vi "PH_BL-Master.PC calc Vac State.vi"(0 "i ref in":refnum<vi>, 2 "Channel Name":string="N/A", 4 "no link":bool, 5 "error in (no error)":errorcluster) -> (14 "i ref out":refnum<vi>, 19 "error out":errorcluster)   [LabVIEW 2014, in "PH_BL-Master.lvlib"]
doc: "This VI sets the vac state to GUI elements and stores it to own attributes."
uses:
  PH_BL-Master.lvlib
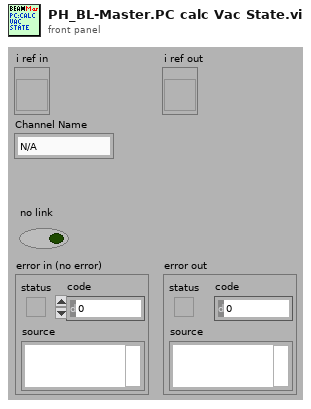
[diagram p1: front panel]
types:
  T1 = typedef "PH_BL-Master.lvlib/PH_BL-Master.i attribute.ctl" = cluster{"Remote controlled":bool, "Boolean Condition Service Subscriber":refnum<vi>[], "Picture Condition Service Subscriber":refnum<vi>[], "R2S":cluster{"GUI Ref":refnum<vi>, "State":bool}, "Vacua":cluster{"GUI Ref":refnum<vi>, "Limit":dbl, "Curr Value":dbl, "in range":bool}[], "O2 Inspection":cluster{"GUI Ref":refnum<vi>, "Concentration":dbl, "State":T2}[], "Boolean Status Service Subscriber":cluster{"GUI Ref":refnum<vi>, "Status":T2, "no Link?":bool, "Status Subscriber Class":T3}[], "Picture Status Service Subscriber":cluster{"GUI Ref":refnum<vi>, "Status":T2, "no Link?":bool, "Status Subscriber Class":T3}[], "6P 4Q Service Subscriber":cluster{"GUI Ref":refnum<vi>, "Selector":T4, "no Link?":bool}[], "Index of latest 6P 4Q changing Instance":i32, "Index of latest Picture Status changing Instance":i32, "Index of latest Boolean Status changing Instance":i32, "Vision ID on same Node":string, "Start Phase over?":bool, "GUI Ref Delete":refnum<vi>}
  T2 = typedef "PH_StatusHandler.lvlib/PH_StatusHandler.Status.ctl" = i16
  T3 = typedef "PH_BL-Master.lvlib/PH_BL-Master.Status Subscriber Class.ctl" = enum16{"unknown", "Switch", "BB", "6P Switch", "Switch GUI", "Switch and 6P State", "Force Sensor"}
  T4 = typedef "PH_4_Pos_Selector.lvlib/PH_4_Pos_Selector.Position Selector.ctl" = u16
  T5 = cluster{"GUI Ref":refnum<vi>, "Limit":dbl, "Curr Value":dbl, "in range":bool}[]
  T6 = cluster{"GUI Ref":refnum<vi>, "Limit":dbl, "Curr Value":dbl, "in range":bool}
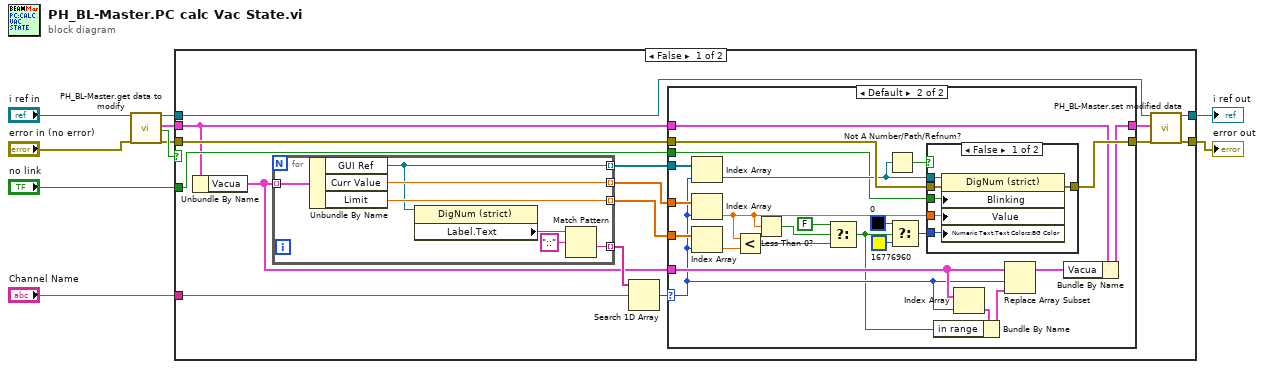
[diagram p0: block diagram]
diagram:
  n1 = call "PH_BL-Master.get data to modify.vi"("i ref in"="i ref in", "error in (no error)"="error in (no error)") -> ("i ref out"=w1:refnum<vi>, "i attribute"=w3:T1, "timed out"=w4:bool, "error out"=w2:errorcluster)  [unwired: 14 in]
  n2 = case shown="False" w4 {
    tunnel: w1 -> [w15 w67]
    tunnel: [w25 w67] -> w9
    tunnel: w2 -> [w23 w66]
    tunnel: [w24 w66] -> w10
    tunnel: w3 -> [w18 _]
    tunnel: "Channel Name" -> [w19 _]
    tunnel: "no link" -> [w21 _]
    frame False {
      n3 = Unbundle By Name(w18) -> ("Vacua"=w14:T5)
      n4 = for {
        tunnel: w14 -> [w65] mode=indexing
        tunnel: [w59] -> w20 mode=indexing
        tunnel: [w64] -> w13 mode=indexing
        tunnel: [w63] -> w12 mode=indexing
        tunnel: [w62] -> w11 mode=indexing
        n5 = Unbundle By Name(w65) -> ("GUI Ref"=w62:refnum<vi>, "Curr Value"=w64:dbl, "Limit"=w63:dbl)
        n6 = property class="DigNum (strict)"(reference=w62) -> ("Label.Text"=w61:string)  [unwired: 1 in, 2 out]
        n7 = Match Pattern(string=w61, regular expression="::") -> (after substring=w59:string)  [unwired: 1 in, 3 out]
      }
      n8 = Search 1D Array(1D array=w20, element=w19) -> (index of element=w16:i32)  [unwired: 1 in]
      n9 = case shown="Default" w16 {
        selector: w16 -> [_ w36]
        tunnel: w23 -> [w26 w51]
        tunnel: [w26 w50] -> w22
        tunnel: w21 -> [_ w34]
        tunnel: w14 -> [_ w37]
        tunnel: w18 -> [w27 w42]
        tunnel: [w27 w41] -> w17
        tunnel: w13 -> [_ w39]
        tunnel: w12 -> [_ w38]
        tunnel: w11 -> [_ w28]
        frame -1 {
        }
        frame Default {
          n10 = Index Array(array=w28, index=w36) -> (element=w44:refnum<vi>)
          n11 = Index Array(array=w39, index=w36) -> (element=w33:dbl)
          n12 = Index Array(array=w38, index=w36) -> (element=w46:dbl)
          n13 = Less?(x=w33, y=w46) -> (x < y?=w30:bool)
          n14 = Less Than 0?(x=w33) -> (x < 0?=w32:bool)
          n15 = Select(t=FALSE, s=w32, f=w30) -> (s? t:f=w29:bool)
          n16 = Not A Number/Path/Refnum?(number/path/refnum=w44) -> (NaN/Path/Refnum?=w45:bool)
          n17 = Select(t=u32 0 ("Color Box"), s=w29, f=u32 16776960 ("Color Box")) -> (s? t:f=w47:u32)
          n18 = case shown="False" w45 {
            tunnel: w44 -> [w57 _]
            tunnel: w51 -> [w56 w58]
            tunnel: [w55 w58] -> w50
            tunnel: w33 -> [w54 _]
            tunnel: w47 -> [w53 _]
            tunnel: w34 -> [w52 _]
            frame False {
              n19 = property class="DigNum (strict)"(reference=w57, error in=w56, "Blinking"=w52, "Value"=w54, "Numeric Text.Text Colors:BG Color"=w53) -> (error out=w55:errorcluster)  [unwired: 1 out]
            }
            frame True {
            }
          }
          n20 = Index Array(array=w37, index=w36) -> (element=w35:T6)
          n21 = Bundle By Name(cluster=w35, "in range"=w29) -> (w40:T6)
          n22 = Replace Array Subset(array=w37, new element=w40, index=w36) -> (w43:T5)
          n23 = Bundle By Name(cluster=w42, "Vacua"=w43) -> (w41:T1)
        }
      }
      n24 = call "PH_BL-Master.set modified data.vi"("i ref in"=w15, "i attribute"=w17, "error in (no error)"=w22) -> ("i ref out"=w25:refnum<vi>, "error out"=w24:errorcluster)  [unwired: 15 in]
    }
    frame True {
    }
  }
  "error out" <- w10
  "i ref out" <- w9
